vi "SDCP SMF Receiver and Transmitter - SMF Rx Table - FGV.vi"(8 "error in (no error)":errorcluster, 9 "Command":enum16{"Reset", "Write", "Read"}(ring), 10 "Bytes in":u8[](array[numeric]), 11 "Parameter descriptors":T2[](array[typedef])) -> (0 "error out":errorcluster, 3 "Elements of log table":T1[](array[typedef]))   [LabVIEW 2020]
uses:
  Typedefs/SDCP - SMF parameter descriptors.ctl
  Typedefs/SDCP - Log Table - Element.ctl
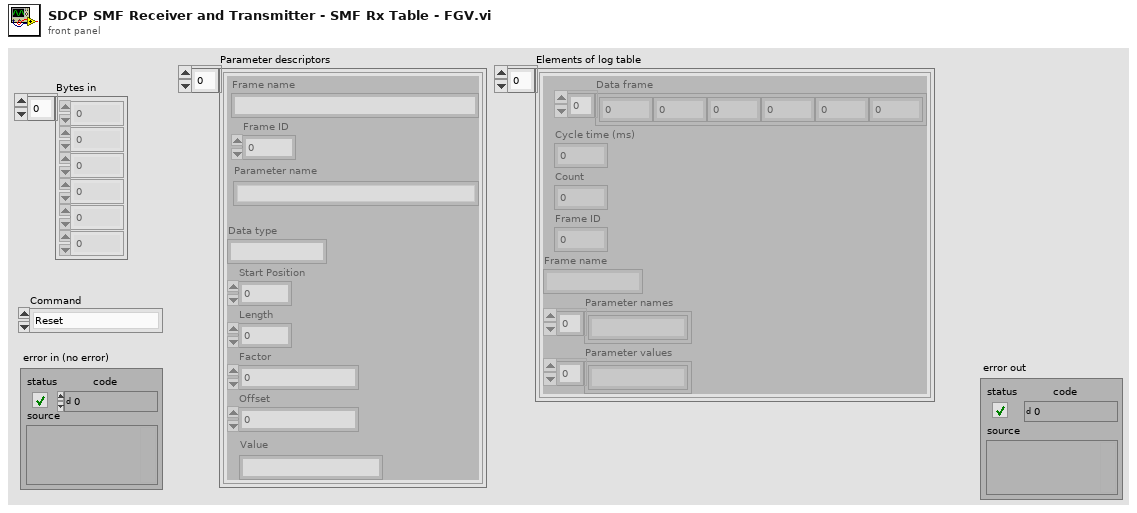
[diagram p1: front panel]
types:
  T1 = typedef "SDCP - Log Table - Element.ctl" = cluster{"Data frame":u8[], "Cycle time (ms)":i32, "Count":i32, "Frame ID":i32, "Frame name":string, "Parameter names":string[], "Parameter values":string[]}
  T2 = typedef "SDCP - SMF parameter descriptors.ctl" = cluster{"Frame name":string, "Frame ID":i32, "Data type":string, "Start Position":i32, "Length":i32, "Factor":dbl, "Offset":dbl, "Parameter name":string, "Value":string}
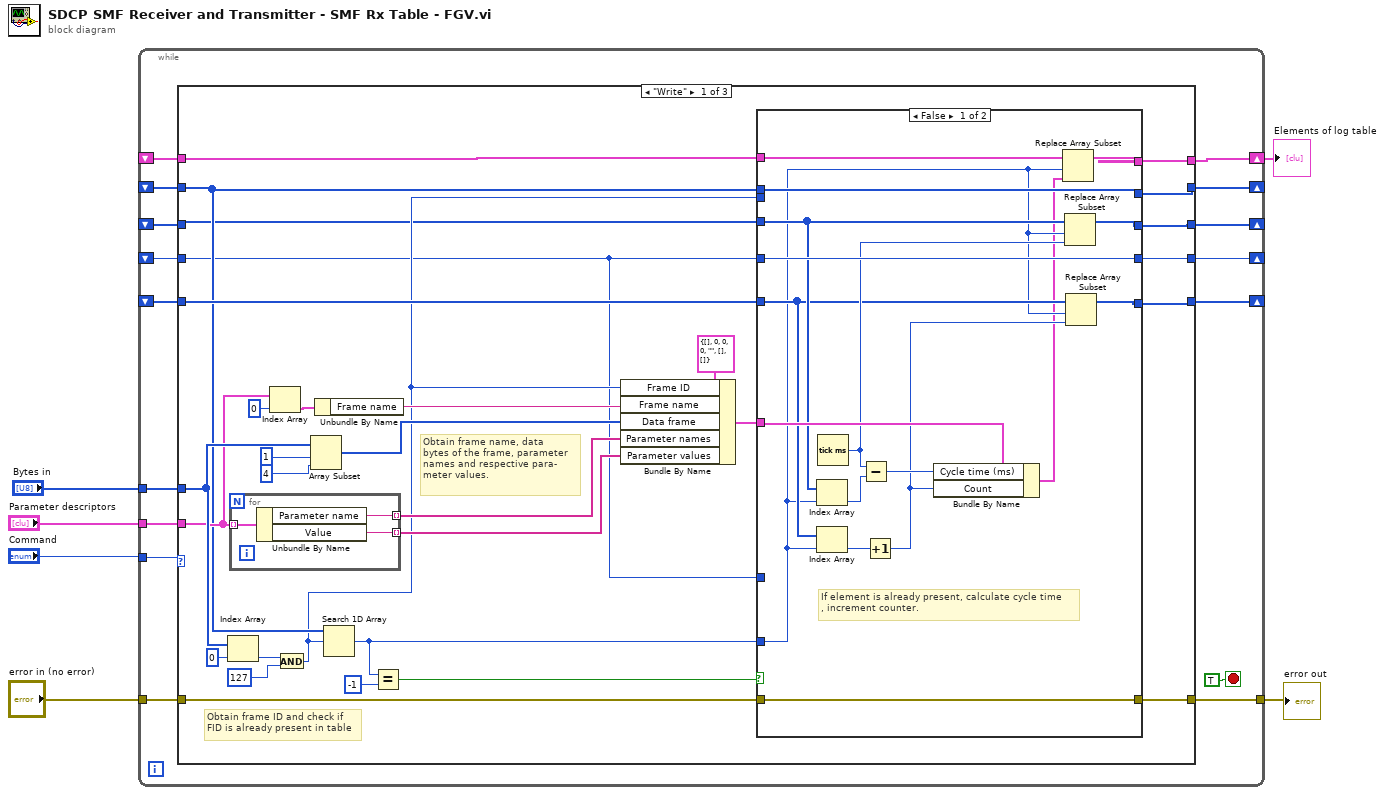
[diagram p0: block diagram]
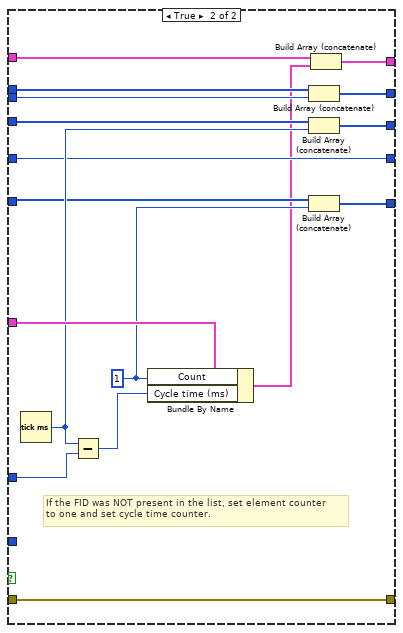
[diagram p2: hidden frame]
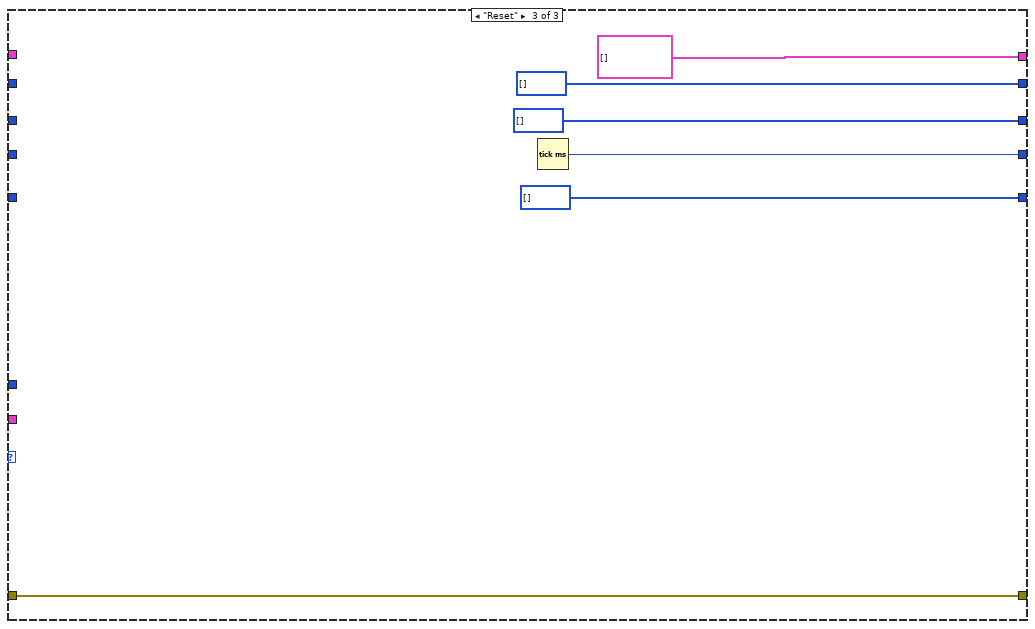
[diagram p4: hidden frame]
diagram:
  n1 = while {
    tunnel: "Command" -> [w21]
    tunnel: "Bytes in" -> [w20]
    tunnel: "Parameter descriptors" -> [w19]
    shift-right: [w17] -> w2
    shift-left: _ -> [w18]
    shift-right: [w16] -> _
    shift-left: _ -> [w15]
    tunnel: "error in (no error)" -> [w14]
    tunnel: [w13] -> w3
    shift-right: [w12] -> _
    shift-left: _ -> [w11]
    shift-right: [w10] -> _
    shift-left: _ -> [w9]
    shift-right: [w8] -> _
    shift-left: _ -> [w7]
    stop <- TRUE stop-if-true
    n2 = case shown="\"Write\"" w21 {
      tunnel: w20 -> [w48 _ _]
      tunnel: w19 -> [w45 _ _]
      tunnel: w18 -> [w35 w96 _]
      tunnel: [w34 w96 T1[] []] -> w17
      tunnel: [w30 w95 u8[] []] -> w16
      tunnel: w15 -> [w32 w95 _]
      tunnel: w14 -> [w37 w91 w100]
      tunnel: [w23 w91 w100] -> w13
      tunnel: [w28 w94 u32[] []] -> w12
      tunnel: w11 -> [w29 w94 _]
      tunnel: [w26 w93 w98] -> w10
      tunnel: w9 -> [w27 w93 _]
      tunnel: [w25 w92 u32[] []] -> w8
      tunnel: w7 -> [w33 w92 _]
      frame "Write" {
        # "Obtain frame name, data\nbytes of the frame, parameter\nnames and respective para-\nmeter values."
        # "Obtain frame ID and check if\nFID is already present in table"
        n3 = Index Array(array=w48, index=0) -> (element=w52:u8)
        n4 = for {
          tunnel: w45 -> [w90] mode=indexing
          tunnel: [w89] -> w40 mode=indexing
          tunnel: [w88] -> w39 mode=indexing
          n5 = Unbundle By Name(w90) -> ("Parameter name"=w89:string, "Value"=w88:string)
        }
        n6 = Index Array(array=w45, index=0) -> (element=w43:T2)
        n7 = And(x=w52, y=u8 127) -> (x .and. y?=w31:u8)
        n8 = Array Subset(array=w48, index=1, length=4) -> (w41:u8[])
        n9 = Unbundle By Name(w43) -> ("Frame name"=w42:string)
        n10 = Search 1D Array(1D array=w32, element=w31) -> (index of element=w24:i32)  [unwired: 1 in]
        n11 = Equal?(x=w24, y=-1) -> (x = y?=w38:bool)
        n12 = Bundle By Name(cluster=T1 {"Data frame"=[], "Cycle time (ms)"=0, "Count"=0, "Frame ID"=0, "Frame name"="", "Parameter names"=[], "Parameter values"=[]} ("SDCP SMF Log Table element"), "Frame ID"=w31, "Frame name"=w42, "Data frame"=w41, "Parameter names"=w40, "Parameter values"=w39) -> (w36:T1)
        n13 = case shown="False" w38 {
          tunnel: w37 -> [w54 w71]
          tunnel: w36 -> [w67 w85]
          tunnel: w35 -> [w69 w87]
          tunnel: [w68 w86] -> w34
          tunnel: w27 -> [_ w84]
          tunnel: w33 -> [w59 w75]
          tunnel: w32 -> [w66 w82]
          tunnel: w31 -> [_ w81]
          tunnel: [w66 w80] -> w30
          tunnel: w29 -> [w62 w79]
          tunnel: [w61 w77] -> w28
          tunnel: w27 -> [w70 w76]
          tunnel: [w70 w76] -> w26
          tunnel: [w58 w74] -> w25
          tunnel: w24 -> [w57 _]
          tunnel: [w54 w71] -> w23
          frame False {
            # "If element is already present, calculate cycle time\n, increment counter."
            n14 = Index Array(array=w62, index=w57) -> (element=w65:u32)
            n15 = Index Array(array=w59, index=w57) -> (element=w63:u32)
            n16 = Tick Count (ms)() -> (millisecond timer value=w60:u32)
            n17 = Subtract(x=w60, y=w65) -> (x-y=w64:u32)
            n18 = Increment(x=w63) -> (x+1=w56:u32)
            n19 = Bundle By Name(cluster=w67, "Cycle time (ms)"=w64, "Count"=w56) -> (w55:T1)
            n20 = Replace Array Subset(array=w69, new element=w55, index=w57) -> (w68:T1[])
            n21 = Replace Array Subset(array=w62, new element=w60, index=w57) -> (w61:u32[])
            n22 = Replace Array Subset(array=w59, new element=w56, index=w57) -> (w58:u32[])
          }
          frame True {
            w73 = 1 ("Count")
            # "If the FID was NOT present in the list, set element counter\nto one and set cycle time counter."
            n23 = Tick Count (ms)() -> (millisecond timer value=w78:u32)
            n24 = Subtract(x=w78, y=w84) -> (x-y=w83:u32)
            n25 = Bundle By Name(cluster=w85, "Count"=w73, "Cycle time (ms)"=w83) -> (w72:T1)
            n26 = Build Array (concatenate)(w82, w81) -> (w80:u8[])
            n27 = Build Array (concatenate)(w79, w78) -> (w77:u32[])
            n28 = Build Array (concatenate)(w75, w73) -> (w74:u32[])
            n29 = Build Array (concatenate)(w87, w72) -> (w86:T1[])
          }
        }
      }
      frame "Read" {
      }
      frame "Reset" {
        n30 = Tick Count (ms)() -> (millisecond timer value=w98:u32)
      }
    }
  }
  "error out" <- w3
  "Elements of log table" <- w2
